vi "R calculator.vi"(10 "Filtered X":dbl[](array[numeric]), 11 "Filtered X 2":dbl[](array[numeric])) -> (3 "Numeric":dbl)   [LabVIEW 2018]
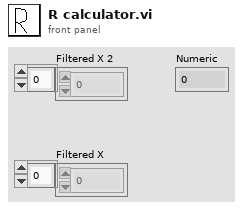
[diagram p1: front panel]
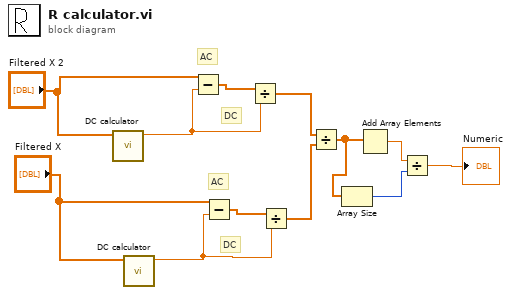
[diagram p0: block diagram]
diagram:
  # "DC"
  # "AC"
  # "DC"
  # "AC"
  n1 = call "DC calculator.vi"("Subset 3"="Filtered X 2") -> ("Numeric"=w3:dbl)  [unwired: 10 in]
  n2 = call "DC calculator.vi"("Subset 3"="Filtered X") -> ("Numeric"=w5:dbl)  [unwired: 10 in]
  n3 = Subtract(x="Filtered X 2", y=w3) -> (x-y=w2:dbl[])
  n4 = Subtract(x="Filtered X", y=w5) -> (x-y=w4:dbl[])
  n5 = Divide(x=w2, y=w3) -> (x/y=w7:dbl[])
  n6 = Divide(x=w4, y=w5) -> (x/y=w8:dbl[])
  n7 = Divide(x=w7, y=w8) -> (x/y=w9:dbl[])
  n8 = Array Size(array=w9) -> (size(s)=w11:i32)
  n9 = Add Array Elements(numeric array=w9) -> (sum=w10:dbl)
  n10 = Divide(x=w10, y=w11) -> (x/y=→"Numeric":dbl)
